vi "Path.vi"() -> (2 "Total":path)   [LabVIEW 2016]
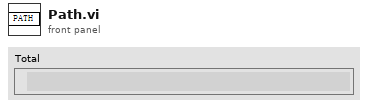
[diagram p1: front panel]
types:
  T1 = enum32{"invalid app kind", "Development System", "Run Time System", "Student Edition", "Embedded LabVIEW", "Evaluation", "Custom"}
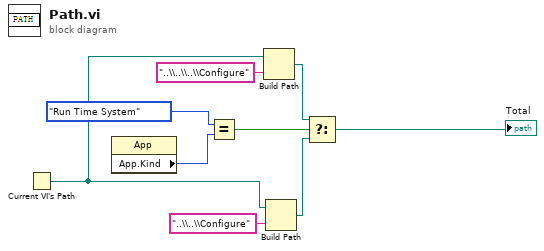
[diagram p0: block diagram]
diagram:
  n1 = Current VI's Path() -> (path=w3:path)
  n2 = property class="App"() -> ("App.Kind"=w9:T1)  [unwired: 2 in, 2 out]
  n3 = Equal?(x=T1."Run Time System" ("应用程序:类别"), y=w9) -> (x = y?=w7:bool)
  n4 = Build Path(base path=w3, name or relative path="..\\..\\..\\Configure" ("名称或相对路径")) -> (appended path=w2:path)
  n5 = Build Path(base path=w3, name or relative path="..\\..\\Configure" ("名称或相对路径")) -> (appended path=w5:path)
  n6 = Select(t=w2, s=w7, f=w5) -> (s? t:f=→"Total":path)
